vi "Get Row and Colum - Single Pixel (SubVI).vi"(8 "Dim":u16=256, 10 "Colum In":u8, 11 "Row In":u8) -> (0 "Last Pixel?":bool, 2 "Colum Out":u8, 3 "Row Out":u8, 6 "Pixel":u16)   [LabVIEW 2017, in "SoC IP Library.lvlib"]
uses:
  SoC IP Library.lvlib
  <vilib>/rvi/FXPMathLib/FxpMul/XNode/nifxpmath_Multiplier.xnode
  <vilib>/rvi/FXPMathLib/sim/FxpSim.dll
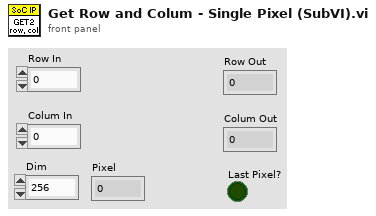
[diagram p1: front panel]
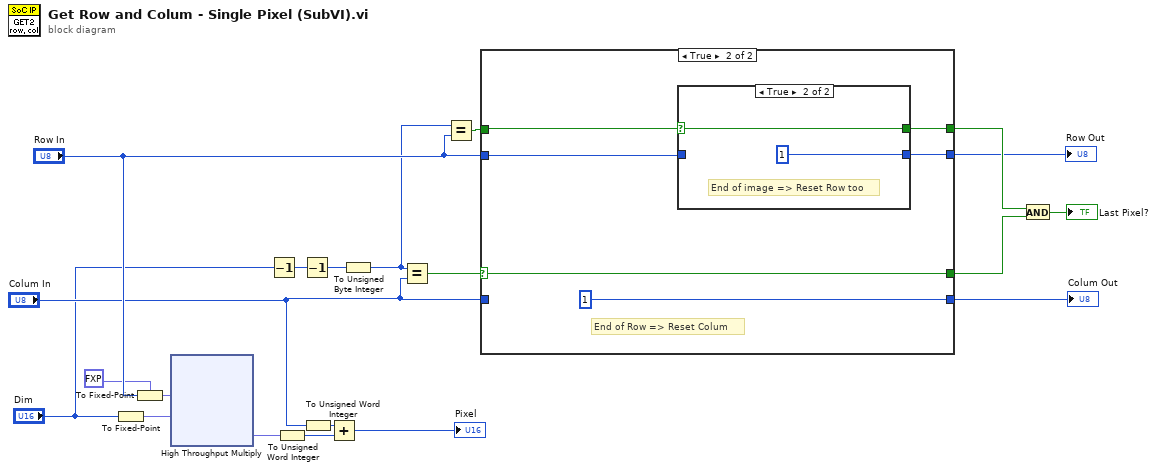
[diagram p0: block diagram]
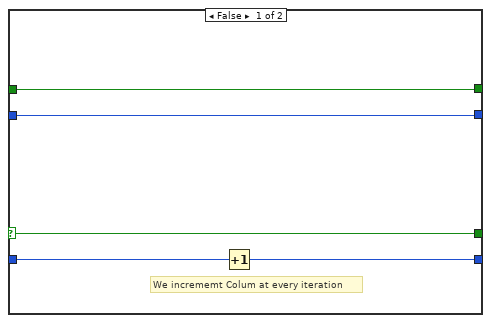
[diagram p2: hidden frame]
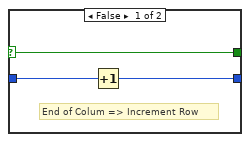
[diagram p3: hidden frame]
diagram:
  n1 = To Fixed-Point(number="Dim") -> (fixed-point=w7:fxp<+,16,16>)  [unwired: 1 in]
  n2 = To Fixed-Point(fixed-point type=fxp<+,8,8> 0.0 ("x"), number="Row In") -> (fixed-point=w8:fxp<+,8,8>)
  n3 = xnode ("High Throughput Multiply")("x"=w8, "y"=w7) -> ("x*y"=w6:fxp<+,16,16>)
  n4 = Decrement(x="Dim") -> (x-1=w12:u16)
  n5 = To Unsigned Word Integer(number=w6) -> (unsigned 16bit integer=w5:u16)
  n6 = Decrement(x=w12) -> (x-1=w11:u16)
  n7 = To Unsigned Word Integer(number="Colum In") -> (unsigned 16bit integer=w3:u16)
  n8 = Add(x=w3, y=w5) -> (x+y=→"Pixel":u16)
  n9 = To Unsigned Byte Integer(number=w11) -> (unsigned 8bit integer=w1:u8)
  n10 = Equal?(x=w1, y="Colum In") -> (x = y?=w20:bool)
  n11 = Equal?(x=w1, y="Row In") -> (x = y?=w15:bool)
  n12 = case shown="True" w20 {
    selector: w20 -> [w23 w30]
    tunnel: [w25 u8 1] -> w19
    tunnel: "Colum In" -> [w24 _]
    tunnel: [w23 w30] -> w18
    tunnel: w15 -> [w21 w29]
    tunnel: "Row In" -> [w22 w26]
    tunnel: [w22 w28] -> w13
    tunnel: [w21 w27] -> w14
    frame False {
      # "We incrememt Colum at every iteration"
      n13 = Increment(x=w24) -> (x+1=w25:u8)
    }
    frame True {
      # "End of Row => Reset Colum"
      n14 = case shown="True" w29 {
        selector: w29 -> [w32 w35]
        tunnel: [w33 u8 1] -> w28
        tunnel: w26 -> [w34 _]
        tunnel: [w32 w35] -> w27
        frame False {
          # "End of Colum => Increment Row"
          n15 = Increment(x=w34) -> (x+1=w33:u8)
        }
        frame True {
          # "End of image => Reset Row too"
        }
      }
    }
  }
  "Row Out" <- w13
  "Colum Out" <- w19
  n16 = And(x=w14, y=w18) -> (x .and. y?=→"Last Pixel?":bool)
